vi "LV to TOML Test.vi"() -> ()   [LabVIEW 2015]
uses:
  lib/TOML.lvlib
panel:
  out "TOML String":string
  in  "Data":T1={"Number"=0.0, "Array"=[[{"Boolean"=FALSE}, {"Boolean"=FALSE}], [{"Boolean"=TRUE}, {"Boolean"=FALSE}]], "Table"={"String"=""}}
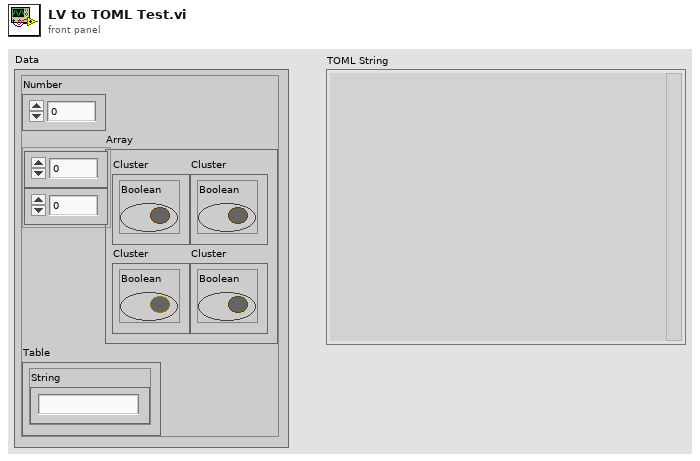
[diagram p1: front panel]
types:
  T1 = cluster{"Number":dbl, "Array":cluster{"Boolean":bool}[][], "Table":cluster{"String":string}}
  T2 = typedef "TOML.lvlib/TOML Value.ctl" = cluster{"\\type":enum16{"Table", "Array", "String", "Integer", "Float", "Boolean", "Offset Date-Time", "Local Date-Time", "Local Date", "Local Time"}, "ÿýÿýÿýÿýÿýÿþÿýÿýÿý\"TOML.lvlib:TOML Key-Value Pair.ctlÿýÿýÿýÿýÿýÿþÿýÿýÿýTOML.lvlib:TOML Value.ctl$$":variant}
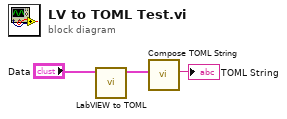
[diagram p0: block diagram]
diagram:
  n1 = call "LabVIEW to TOML.vi"("LV Value"="Data") -> ("TOML Value"=w2:T2)  [unwired: 9 in, 1 out]
  n2 = call "Compose TOML String.vi"("Value"=w2) -> ("String"=→"TOML String":string)  [unwired: 10 in]
